vi "Run Ramped Cascade.vi"(9 "Reset?":bool=TRUE, 10 "Griddy Command":T6, 11 "Cascade In":T1) -> (2 "Finished?":bool, 3 "Cascade Out":T1={"DeviceStatus"={"status"=FALSE, "code"=0, "source"=""}, "Type"=enum."PWM", "PWM"={"PWM Channel"=enum."Invalid", "DeadBand"={"Name"="", "maxPositivePwm"=0, "minPositivePwm"=0, "centerPwm"=0, "maxNegativePwm"=0, "minNegativePwm"=0, "angularRange"=0}}, "CAN"={"Device Number"=0, "SetOutput VI Ref"=variant, "GetOutput VI Ref"=variant, "Enable VI Ref"=variant, "Disable VI Ref"=variant, "Data"=variant}, "Invert"=FALSE, "DIO PWM"={"PWM \"Enable\" Channel"=enum."Invalid", "DIOChannel"=enum."Invalid", "PWM Rate"=0.0}})   [LabVIEW 2020]
uses:
  Typedefs/Teleop Manipulator Commands.ctl
  <vilib>/Rock Robotics/WPI/MotorControl/WPI_MotorControlDeviceRef.ctl
  <vilib>/Rock Robotics/WPI/MotorControl/WPI_MotorControlType.ctl
  <vilib>/Rock Robotics/SystemInterfaces/DIO/FPGA_DIOPWMChannel.ctl
  <vilib>/Rock Robotics/WPI/PWM/WPI_PWMDeadband.ctl
  <vilib>/Rock Robotics/SystemInterfaces/DIO/FPGA_DIOChannel.ctl
  <vilib>/Rock Robotics/WPI/ThirdParty/REV Robotics/REVLib/Typedef/Spark MAX Control Type.ctl
  66668532-1734-44c2-abcf-6a6552019c3d.vi
  <vilib>/Comparison/Less/Less Functor/Less Functor.lvclass
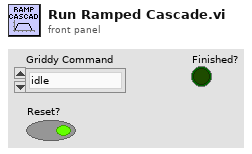
[diagram p1: front panel]
types:
  T1 = typedef "WPI_MotorControlDeviceRef.ctl" = cluster{"DeviceStatus":errorcluster, "Type":T2, "PWM":cluster{"PWM Channel":T3, "DeadBand":T4}, "CAN":cluster{"Device Number":u8, "SetOutput VI Ref":variant, "GetOutput VI Ref":variant, "Enable VI Ref":variant, "Disable VI Ref":variant, "Data":variant}, "Invert":bool, "DIO PWM":cluster{"PWM \"Enable\" Channel":T3, "DIOChannel":T5, "PWM Rate":dbl}}
  T2 = typedef "WPI_MotorControlType.ctl" = enum16{"PWM", "CAN", "DIO PWM"}
  T3 = typedef "FPGA_DIOPWMChannel.ctl" = enum8{"PWM 0", "PWM 1", "PWM 2", "PWM 3", "PWM 4", "PWM 5", "PWM 6", "PWM 7", "PWM 8", "PWM 9", "PWM MXP 0", "PWM MXP 1", "PWM MXP 2", "PWM MXP 3", "PWM MXP 4", "PWM MXP 5", "PWM MXP 6", "PWM MXP 7", "PWM MXP 8", "PWM MXP 9", "Invalid"}
  T4 = typedef "WPI_PWMDeadband.ctl" = cluster{"Name":string, "maxPositivePwm":i32, "minPositivePwm":i32, "centerPwm":i32, "maxNegativePwm":i32, "minNegativePwm":i32, "angularRange":u16}
  T5 = typedef "FPGA_DIOChannel.ctl" = enum8{"DIO 0", "DIO 1", "DIO 2", "DIO 3", "DIO 4", "DIO 5", "DIO 6", "DIO 7", "DIO 8", "DIO 9", "DIO MXP 0", "DIO MXP 1", "DIO MXP 2", "DIO MXP 3", "DIO MXP 4", "DIO MXP 5", "DIO MXP 6", "DIO MXP 7", "DIO MXP 8", "DIO MXP 9", "DIO MXP 10", "DIO MXP 11", "DIO MXP 12", "DIO MXP 13", "DIO MXP 14", "DIO MXP 15", "SPI Port CS1", "SPI Port CS2", "SPI Port CS3", "SPI Port MISO", "SPI Port MOSI", "Invalid"}
  T6 = typedef "Teleop Manipulator Commands.ctl" = enum16{"idle", "intake cone sideways", "intake cone upright", "intake cone feeder", "intake cube feeder", "intake cube", "score low cone", "score low cube", "score mid cone", "score mid cube", "score high cone", "score high cube", "score mid cone up"}
  T7 = cluster{string, "Starting Position":dbl, "Preset in Use?":bool, "more Velocity values--scary":dbl[]}[]
  T8 = cluster{"Safe Wrist Position":dbl, "Margin of Error":cluster{"Safety Wrist Margin":dbl, "Cascade Margin":dbl, "Final Wrist Margin":dbl}, "grid-dy":cluster{"Griddy Preset":string, "cascade pos":dbl, "wrist pos":dbl, "Overrides":cluster{"Margin of Error Overrides":cluster{"Safety Wrist Margin":dbl, "Cascade Margin":dbl, "Final Wrist Margin":dbl}, "Override?":bool}}[]}
  T9 = cluster{string, "Starting Position":dbl, "Preset in Use?":bool, "Velocity Profile":dbl[]}[]
  T10 = cluster{"Safety Wrist Margin":dbl, "Cascade Margin":dbl, "Final Wrist Margin":dbl}
  T11 = cluster{"Griddy Preset":string, "cascade pos":dbl, "wrist pos":dbl, "Overrides":cluster{"Margin of Error Overrides":cluster{"Safety Wrist Margin":dbl, "Cascade Margin":dbl, "Final Wrist Margin":dbl}, "Override?":bool}}[]
  T12 = cluster{"Griddy Preset":string, "cascade pos":dbl, "wrist pos":dbl, "Overrides":cluster{"Margin of Error Overrides":cluster{"Safety Wrist Margin":dbl, "Cascade Margin":dbl, "Final Wrist Margin":dbl}, "Override?":bool}}
  T13 = cluster{string, "Starting Position":dbl, "Preset in Use?":bool, "more Velocity values--scary":dbl[]}
  T14 = cluster{string, "Starting Position":dbl, "Preset in Use?":bool, "Velocity Profile":dbl[]}
  T15 = typedef "Spark MAX Control Type.ctl" = enum16{"Percent VBus", "Voltage", "Velocity", "Position", "Smart Motion", "Current", "Smart Velocity"}
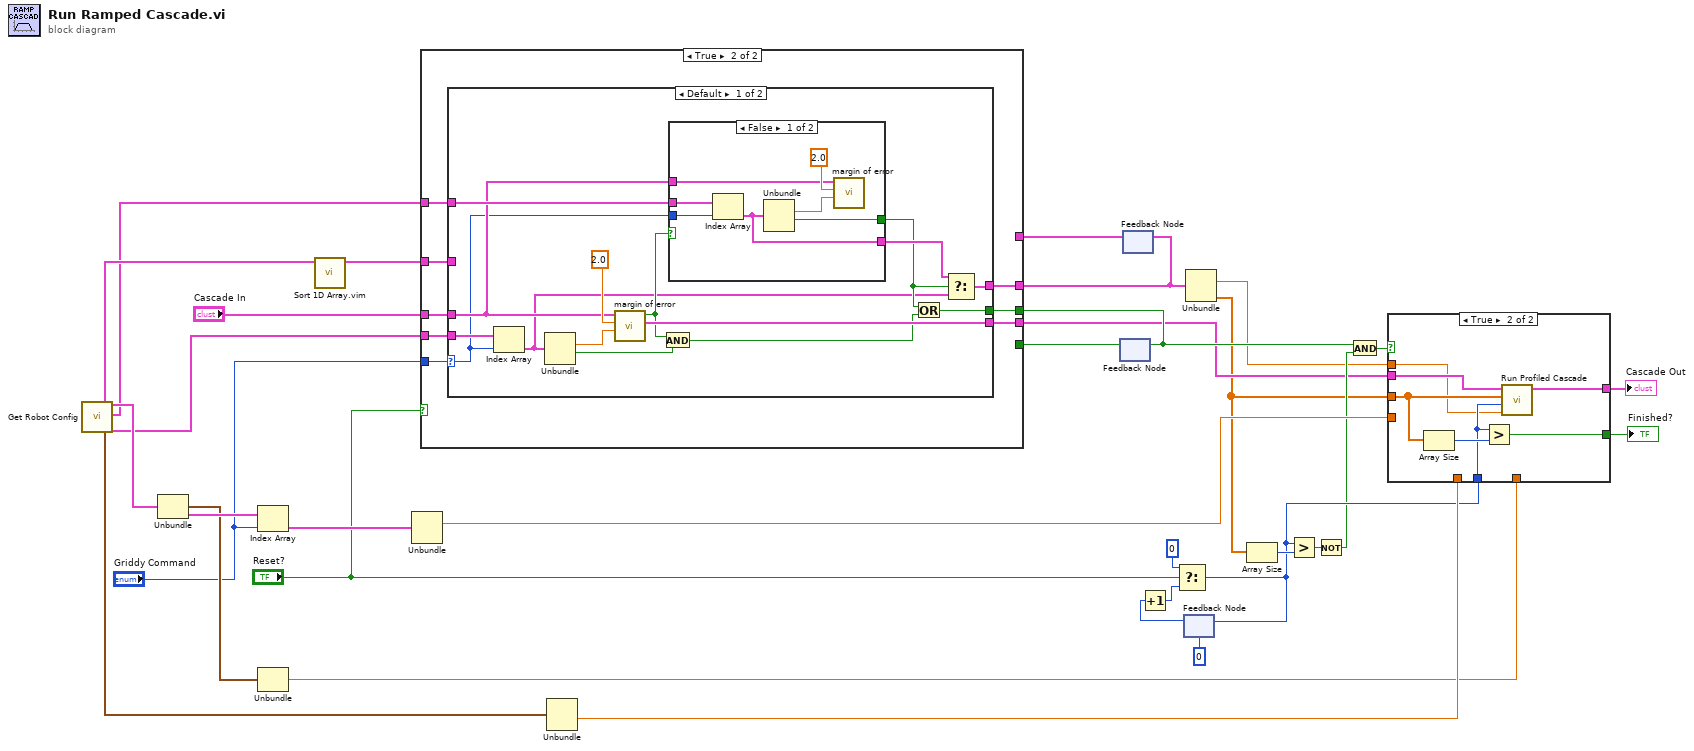
[diagram p0: block diagram]
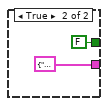
[diagram p3: hidden frame]
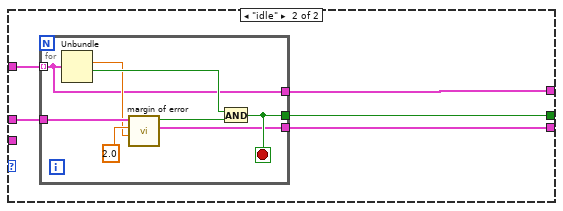
[diagram p4: hidden frame]
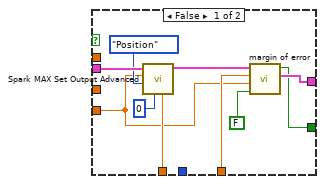
[diagram p5: hidden frame]
diagram:
  n1 = call "Get Robot Config.vi"() -> ("Idle Ramping Table"=w2:T7, "Cascade FeedForward Constants"=w25:cluster{"kA":dbl, "kS":dbl, "kG":dbl, "kV":dbl}, "Manipulator Config"=w28:T8, "Scoring Overrides Ramping Table"=w1:T7, "Score Ramping Table"=w14:T9)  [unwired: 12 in, 3 out]
  n2 = Unbundle(w28) -> ("Margin of Error"=w21:T10, "grid-dy"=w27:T11)  [unwired: 1 out]
  n3 = Index Array(array=w27, index="Griddy Command") -> (element=w26:T12)
  n4 = Unbundle(w21) -> ("Cascade Margin"=w20:dbl)  [unwired: 2 out]
  n5 = call "Sort 1D Array.vim"("unsorted array"=w2) -> ("sorted array"=w33:T7)  [unwired: 10 in]
  n6 = Unbundle(w26) -> ("cascade pos"=w32:dbl)  [unwired: 3 out]
  n7 = Unbundle(w25) -> ("kG"=w24:dbl)  [unwired: 3 out]
  n8 = feedback #1() -> (w12:bool)  [unwired: 1 in]
  n9 = feedback #2() -> (w11:T13)  [unwired: 1 in]
  n10 = case shown="True" "Reset?" {
    tunnel: w33 -> [_ w44]
    tunnel: "Cascade In" -> [w36 w43]
    tunnel: "Griddy Command" -> [_ w42]
    tunnel: w14 -> [_ w41]
    tunnel: [w36 w40] -> w4
    tunnel: [w34 w39] -> w6
    tunnel: [w35 w38] -> w7
    tunnel: w12 -> [w35 _]
    tunnel: w11 -> [w34 _]
    tunnel: w1 -> [_ w37]
    frame False {
    }
    frame True {
      n11 = case shown="Default" w42 {
        selector: w42 -> [w45 _]
        tunnel: w44 -> [_ w73]
        tunnel: w43 -> [w52 w72]
        tunnel: w41 -> [w59 _]
        tunnel: [w56 w71] -> w40
        tunnel: [w51 w70] -> w38
        tunnel: [w49 w69] -> w39
        tunnel: w37 -> [w54 _]
        frame Default {
          n12 = Index Array(array=w59, index=w45) -> (element=w46:T14)
          n13 = Unbundle(w46) -> ("Starting Position"=w57:dbl, "Preset in Use?"=w55:bool)  [unwired: 2 out]
          n14 = call "margin of error.vi"("setpoint"=w57, "margin of error"=2.0, "Motor In"=w52) -> ("Motor Out"=w56:T1, "In Range?"=w53:bool)  [unwired: 7 in]
          n15 = And(x=w53, y=w55) -> (x .and. y?=w50:bool)
          n16 = case shown="False" w53 {
            tunnel: w54 -> [w63 _]
            tunnel: w52 -> [w64 _]
            tunnel: [w62 FALSE] -> w47
            tunnel: [w61 T13 {"", "Starting Position"=0.0, "Preset in Use?"=FALSE, "more Velocity values--scary"=[]} ("Profiled Preset")] -> w48
            tunnel: w45 -> [w60 _]
            frame False {
              n17 = Index Array(array=w63, index=w60) -> (element=w61:T13)
              n18 = Unbundle(w61) -> ("Starting Position"=w66:dbl, "Preset in Use?"=w62:bool)  [unwired: 2 out]
              n19 = call "margin of error.vi"("setpoint"=w66, "margin of error"=2.0, "Motor In"=w64) -> ()  [unwired: 7 in, 2 out]
            }
            frame True {
            }
          }
          n20 = Or(x=w47, y=w50) -> (x .or. y?=w51:bool)
          n21 = Select(t=w48, s=w47, f=w46) -> (s? t:f=w49:T14)
        }
        frame "idle" {
          n22 = for {
            tunnel: w73 -> [w74] mode=indexing
            tunnel: [w80] -> w70
            tunnel: [w74] -> w69
            tunnel: w72 -> [w79]
            tunnel: [w75] -> w71
            stop <- w80 stop-if-true
            n23 = Unbundle(w74) -> ("Starting Position"=w77:dbl, "Preset in Use?"=w81:bool)  [unwired: 2 out]
            n24 = call "margin of error.vi"("setpoint"=w77, "margin of error"=2.0, "Motor In"=w79) -> ("Motor Out"=w75:T1, "In Range?"=w76:bool)  [unwired: 7 in]
            n25 = And(x=w81, y=w76) -> (x .and. y?=w80:bool)
          }
        }
      }
    }
  }
  n26 = feedback-in #1(w7) -> ()
  n27 = feedback-in #2(w6) -> ()
  n28 = feedback #3(0) -> (w22:i32)
  n29 = Increment(x=w22) -> (x+1=w23:i32)
  n30 = Select(t=0, s="Reset?", f=w23) -> (s? t:f=w17:i32)
  n31 = feedback-in #3(w17) -> ()
  n32 = Unbundle(w6) -> ("Starting Position"=w5:dbl, "more Velocity values--scary"=w3:dbl[])  [unwired: 2 out]
  n33 = Array Size(array=w3) -> (size(s)=w18:i32)
  n34 = Greater?(x=w17, y=w18) -> (0:w16:bool)
  n35 = Not(x=w16) -> (.not. x?=w8:bool)
  n36 = And(x=w7, y=w8) -> (x .and. y?=w9:bool)
  n37 = case shown="True" w9 {
    tunnel: w3 -> [_ w96]
    tunnel: w4 -> [w91 w98]
    tunnel: w32 -> [w82 _]
    tunnel: w17 -> [_ w94]
    tunnel: [w86 w97] -> w29
    tunnel: w24 -> [w88 _]
    tunnel: [w85 w93] -> w19
    tunnel: w20 -> [w83 _]
    tunnel: w5 -> [_ w92]
    frame False {
      n38 = call <vilib>:"Spark MAX Set Output Advanced.vi"("Arbitrary Feed Forward (0)"=w88, "PIDF Slot (0)"=0, "Control Mode"=Spark_MAX_Control_Type."Position", "Setpoint"=w82, "MotorControlDevRef"=w91) -> ("MotorControlDevRef"=w87:T1)  [unwired: 5 in, 1 out]
      n39 = call "margin of error.vi"("Wrist Motor?"=FALSE, "setpoint"=w82, "margin of error"=w83, "Motor In"=w87) -> ("Motor Out"=w86:T1, "In Range?"=w85:bool)  [unwired: 6 in]
    }
    frame True {
      n40 = Array Size(array=w96) -> (size(s)=w95:i32)
      n41 = Greater?(x=w94, y=w95) -> (0:w93:bool)
      n42 = call "Run Profiled Cascade.vi"("Cascade Start Position"=w92, "Iteration"=w94, "Velocity Profile"=w96, "Cascade In"=w98) -> ("Cascade Out"=w97:T1)  [unwired: 7 in]
    }
  }
  "Cascade Out" <- w29
  "Finished?" <- w19
